vi "Write Default Value.vi"(10 "Data":string, 11 "Channel in":refnum<class "TBM channel.lvclass">) -> (3 "Channel out":refnum<class "TBM channel.lvclass">)   [LabVIEW 2015, in "PID Module 2 configuration.lvclass"]
uses:
  PID Module 2 configuration.lvclass
  <vilib>/NI/Tag Bus Module Framework/channel/TBM channel.lvclass
  <vilib>/NI/Tag Bus/tag/default value polymorphs/write default value Double.vi
  <vilib>/NI/Tag Bus/tag/tag descriptor.lvclass
panel:
  out "error out":errorcluster
  in  "error in":errorcluster
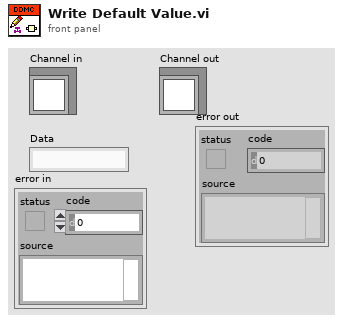
[diagram p1: front panel]
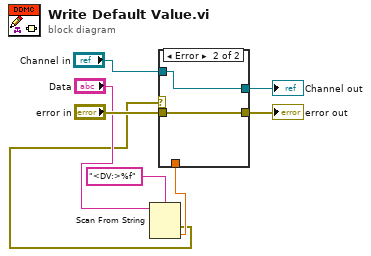
[diagram p0: block diagram]
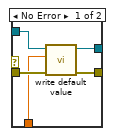
[diagram p2: hidden frame]
diagram:
  n1 = Scan From String(format string="<DV:>%f", input string="Data") -> (error out=w1:errorcluster, output 1=w2:dbl)  [unwired: 3 in, 2 out]
  n2 = case shown="Error" w1 {
    tunnel: "Channel in" -> [w13 w15]
    tunnel: [w12 w15] -> w7
    tunnel: "error in" -> [w11 w14]
    tunnel: [w10 w14] -> w5
    tunnel: w2 -> [w9 _]
    frame No Error {
      n3 = call-poly <vilib>:"write default value.vi"("error in"=w11, "default value"=w9, "system tag in"=w13) -> ("error out"=w10:errorcluster, "system tag out"=w12:refnum<class "TBM channel.lvclass">)  [unwired: 7 in]
    }
    frame Error {
    }
  }
  "Channel out" <- w7
  "error out" <- w5
